vi "Main_良率計算.vi"() -> (1 "total良率":dbl, 2 "output cluster 2":T2, 3 "Cluster 6":T1)   [LabVIEW 2019]
uses:
  LLB/Commonly VI/Main Glb.vi
  LLB/Commonly VI.lvlib
panel:
  out "Total 良率 3":dbl
  in  "Cluster 5":T2
  out "output cluster":T1
  out "S7 焊接次數":u16
  in  "Cluster 4":T1
  out "S12 預留_26":i32
  out "總投入數量":i32
  out "S15 良品出料數量":i32
  out "S13 NG排出數量":i32
  out "S12熱熔次數":i32
  out "S11 測高良率":dbl
  out "S3 Format良率":dbl
  out "S3 Program良率":dbl
  out "S4 電壓良率":dbl
  out "S4 Scan良率":dbl
  out "S2 測電流良率":dbl
  out "S2 Programt良率":dbl
  out "S2 Format良率":dbl
  out "條碼良率":dbl
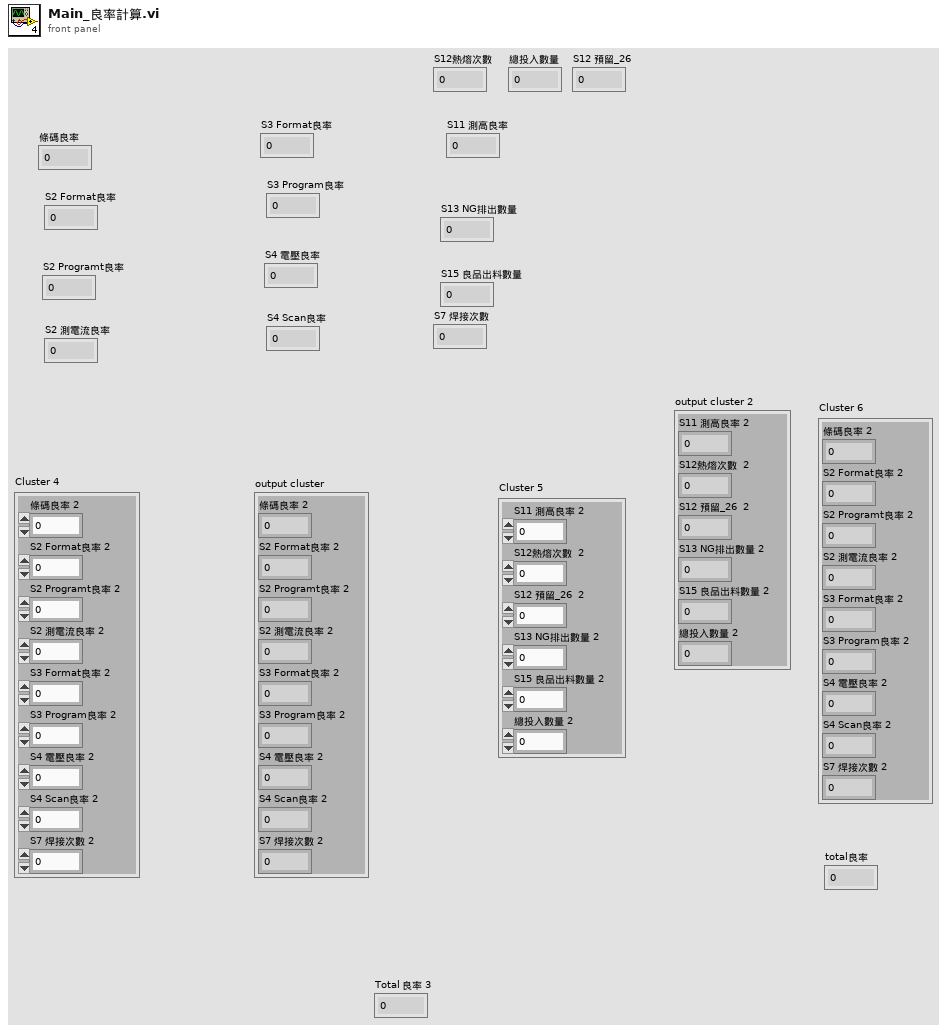
[diagram p1: front panel]
types:
  T1 = cluster{"條碼良率 2":dbl, "S2 Format良率 2":dbl, "S2 Programt良率 2":dbl, "S2 測電流良率 2":dbl, "S3 Format良率 2":dbl, "S3 Program良率 2":dbl, "S4 電壓良率 2":dbl, "S4 Scan良率 2":dbl, "S7 焊接次數 2":i32}
  T2 = cluster{"S11 測高良率 2":dbl, "S12熱熔次數  2":i32, "S12 預留_26  2":i32, "S13 NG排出數量 2":i32, "S15 良品出料數量 2":i32, "總投入數量 2":i32}
  T3 = typedef "良率計算.ctl" = enum16{"條碼OK_0", "條碼NG_1", "S2 format OK_2", "S2 format NG_3", "S2 program OK_4", "S2 program NG_5", "S2 測電流OK_6", "S2 測電流NG_7", "S3 format OK_8", "S3 format NG_9", "S3 program OK_10", "S3 program NG_11", "S4 測電壓OK_12", "S4 測電壓NG_13", "S4 Scan OK_14", "S4 Scan NG_15", "S4 預留_16", "S4 預留_17", "S7 焊接次數_17", "S7 預留_19", "S10 預留_20", "S10 預留_21", "S11 預留_22", "S11 雷射測高OK_23", "S11 雷射測高NG_24", "S12 熱熔次數_25", "S12 預留_26", "S13 NG排出數量_27", "S15 良品出料數量_28", "總投入數量_29"}
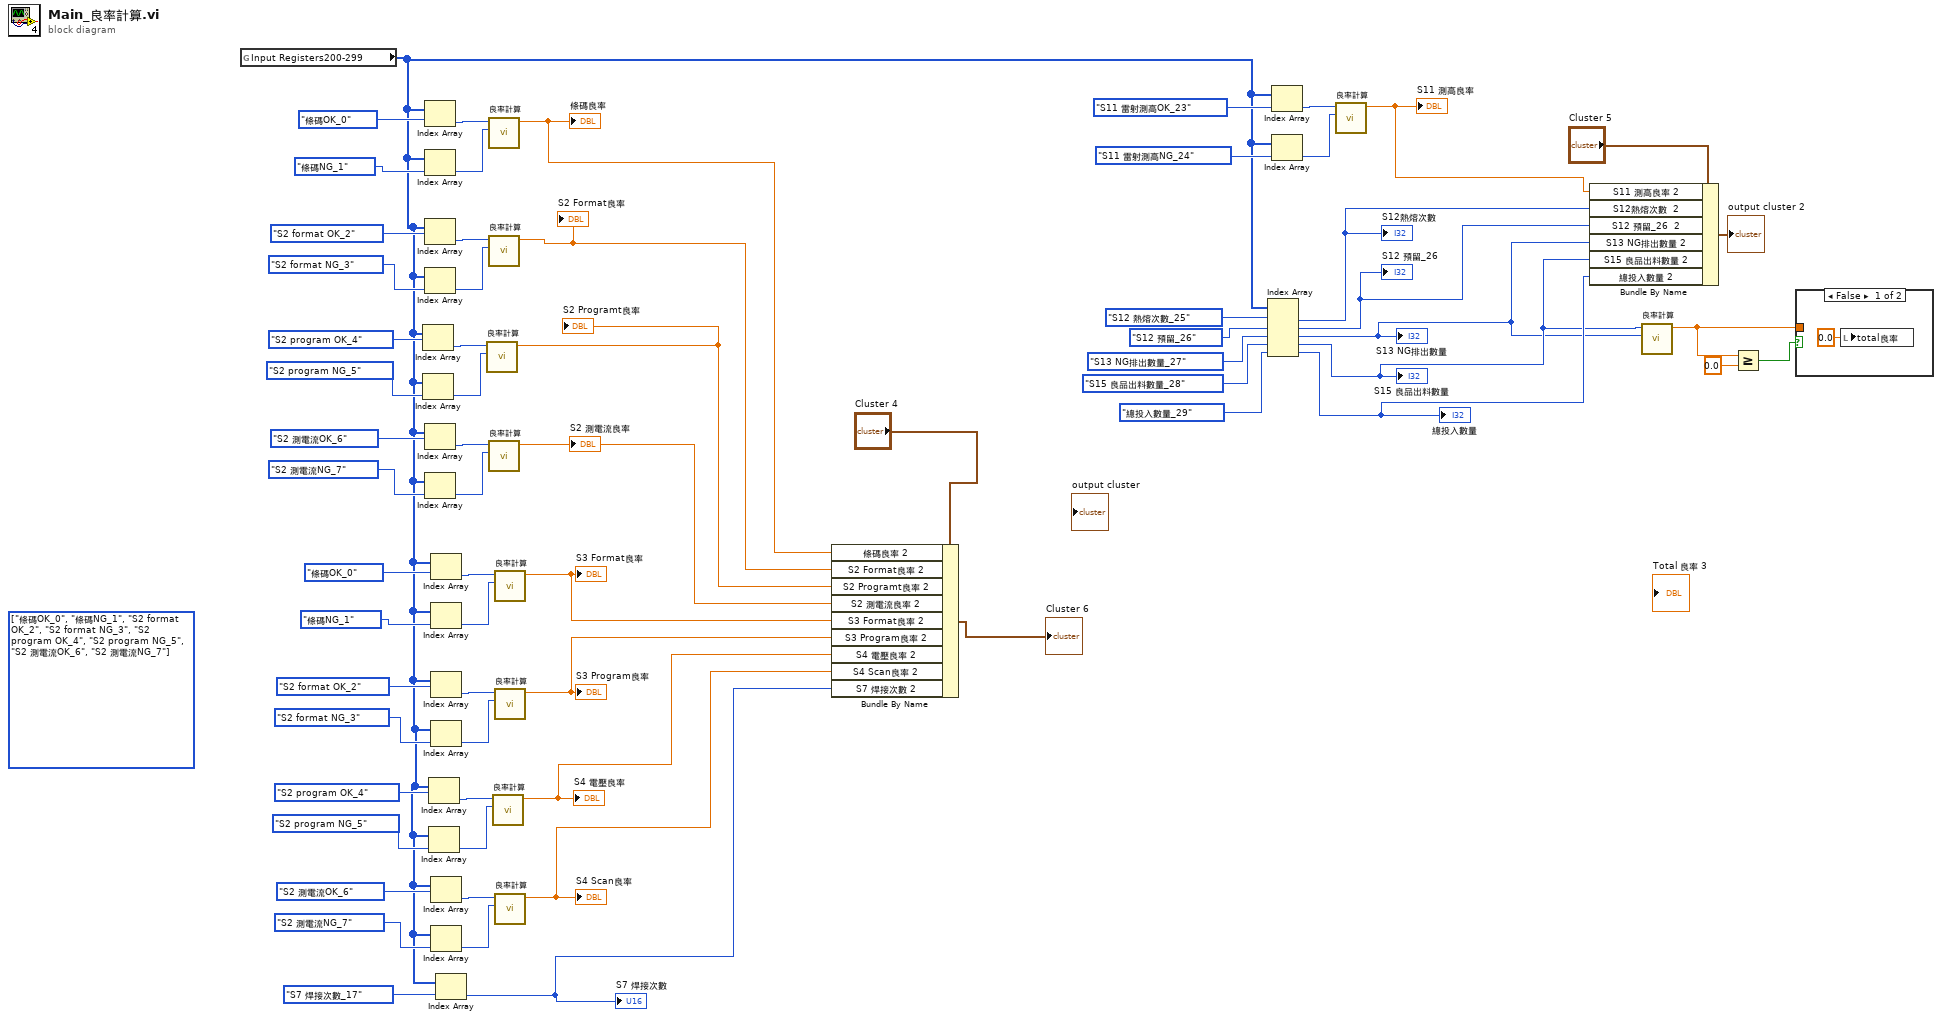
[diagram p0: block diagram]
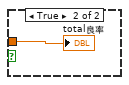
[diagram p2: hidden frame]
diagram:
  (unwired) T3[] [enum."條碼OK_0", enum."條碼NG_1", enum."S2 format OK_2", enum."S2 format NG_3", enum."S2 program OK_4", enum."S2 program NG_5", enum."S2 測電流OK_6", enum."S2 測電流NG_7"] items=["條碼OK_0", "條碼NG_1", "S2 format OK_2", "S2 format NG_3", "S2 program OK_4", "S2 program NG_5", "S2 測電流OK_6", "S2 測電流NG_7", "S3 format OK_8", "S3 format NG_9", "S3 program OK_10", "S3 program NG_11", "S4 測電壓OK_12", "S4 測電壓NG_13", "S4 Scan OK_14", "S4 Scan NG_15", "S4 預留_16", "S4 預留_17", "S7 焊接次數_17", "S7 預留_19", "S10 預留_20", "S10 預留_21", "S11 預留_22", "S11 雷射測高OK_23", "S11 雷射測高NG_24", "S12 熱熔次數_25", "S12 預留_26", "S13 NG排出數量_27", "S15 良品出料數量_28", "總投入數量_29"]
  n1 = global read "Main Glb.vi" "Input Registers200-299"() -> (w7:u16[])
  n2 = Index Array(array=w7, index=良率計算."S2 program OK_4") -> (element=w57:u16)
  n3 = Index Array(array=w7, index=良率計算."S2 program NG_5") -> (element=w56:u16)
  n4 = Index Array(array=w7, index=良率計算."條碼OK_0") -> (element=w65:u16)
  n5 = Index Array(array=w7, index=良率計算."條碼NG_1") -> (element=w64:u16)
  n6 = Index Array(array=w7, index=良率計算."S2 format OK_2") -> (element=w58:u16)
  n7 = Index Array(array=w7, index=良率計算."S2 format NG_3") -> (element=w59:u16)
  n8 = Index Array(array=w7, index=良率計算."S2 測電流OK_6") -> (element=w50:u16)
  n9 = Index Array(array=w7, index=良率計算."S2 測電流NG_7") -> (element=w51:u16)
  n10 = Index Array(array=w7, index=良率計算."S2 program OK_4") -> (element=w42:u16)
  n11 = Index Array(array=w7, index=良率計算."S2 program NG_5") -> (element=w43:u16)
  n12 = Index Array(array=w7, index=良率計算."條碼OK_0") -> (element=w34:u16)
  n13 = Index Array(array=w7, index=良率計算."條碼NG_1") -> (element=w35:u16)
  n14 = Index Array(array=w7, index=良率計算."S2 format OK_2") -> (element=w41:u16)
  n15 = Index Array(array=w7, index=良率計算."S2 format NG_3") -> (element=w40:u16)
  n16 = Index Array(array=w7, index=良率計算."S2 測電流OK_6") -> (element=w49:u16)
  n17 = Index Array(array=w7, index=良率計算."S2 測電流NG_7") -> (element=w48:u16)
  n18 = Index Array(array=w7, index=良率計算."S7 焊接次數_17") -> (element=w14:u16)
  "S7 焊接次數" <- w14
  n19 = call "良率計算.vi"("NG"=w56, "OK"=w57) -> ("良率"=w20:dbl)  [unwired: 9 in]
  "S2 Programt良率" <- w20
  n20 = call "良率計算.vi"("NG"=w64, "OK"=w65) -> ("良率"=w23:dbl)  [unwired: 9 in]
  "條碼良率" <- w23
  n21 = call "良率計算.vi"("NG"=w59, "OK"=w58) -> ("良率"=w21:dbl)  [unwired: 9 in]
  "S2 Format良率" <- w21
  n22 = call "良率計算.vi"("NG"=w51, "OK"=w50) -> ("良率"=w19:dbl)  [unwired: 9 in]
  "S2 測電流良率" <- w19
  n23 = call "良率計算.vi"("NG"=w43, "OK"=w42) -> ("良率"=w16:dbl)  [unwired: 9 in]
  "S4 電壓良率" <- w16
  n24 = call "良率計算.vi"("NG"=w35, "OK"=w34) -> ("良率"=w18:dbl)  [unwired: 9 in]
  "S3 Format良率" <- w18
  n25 = call "良率計算.vi"("NG"=w40, "OK"=w41) -> ("良率"=w17:dbl)  [unwired: 9 in]
  "S3 Program良率" <- w17
  n26 = call "良率計算.vi"("NG"=w48, "OK"=w49) -> ("良率"=w15:dbl)  [unwired: 9 in]
  "S4 Scan良率" <- w15
  n27 = Bundle By Name(cluster="Cluster 4", "條碼良率 2"=w23, "S2 Format良率 2"=w21, "S2 Programt良率 2"=w20, "S2 測電流良率 2"=w19, "S3 Format良率 2"=w18, "S3 Program良率 2"=w17, "S4 電壓良率 2"=w16, "S4 Scan良率 2"=w15, "S7 焊接次數 2"=w14) -> (→"Cluster 6":T1)
  n28 = Index Array(array=w7, index #1=良率計算."S12 熱熔次數_25", index #2=良率計算."S12 預留_26", index #3=良率計算."S13 NG排出數量_27", index #4=良率計算."S15 良品出料數量_28", index #5=良率計算."總投入數量_29") -> (element #1=w10:u16, element #2=w9:u16, element #3=w4:u16, element #4=w5:u16, element #5=w8:u16)
  "S12熱熔次數" <- w10
  "S13 NG排出數量" <- w4
  "S15 良品出料數量" <- w5
  "總投入數量" <- w8
  "S12 預留_26" <- w9
  n29 = Index Array(array=w7, index=良率計算."S11 雷射測高OK_23") -> (element=w32:u16)
  n30 = Index Array(array=w7, index=良率計算."S11 雷射測高NG_24") -> (element=w31:u16)
  n31 = call "良率計算.vi"("NG"=w31, "OK"=w32) -> ("良率"=w11:dbl)  [unwired: 9 in]
  "S11 測高良率" <- w11
  n32 = Bundle By Name(cluster="Cluster 5", "S11 測高良率 2"=w11, "S12熱熔次數  2"=w10, "S12 預留_26  2"=w9, "S13 NG排出數量 2"=w4, "S15 良品出料數量 2"=w5, "總投入數量 2"=w8) -> (→"output cluster 2":T2)
  n33 = call "良率計算.vi"("NG"=w4, "OK"=w5) -> ("良率"=w2:dbl)  [unwired: 9 in]
  n34 = Greater Or Equal?(x=w2, y=0.0) -> (x >= y?=w1:bool)
  n35 = case shown="False" w1 {
    tunnel: w2 -> [_ w67]
    frame False {
      n36 = local write "total良率"(0.0 ("total良率")) -> ()
    }
    frame True {
      "total良率" <- w67
    }
  }
